vi "Launcher.vi"(8 "Error in (no error)":errorcluster) -> (0 "Error out":errorcluster)   [LabVIEW 2021]
uses:
  Controller/Controller/Controller.lvclass
  C:/Program Files/National Instruments/LabVIEW 2021/vi.lib/ActorFramework/Actor/Actor.lvclass
  <vilib>/ActorFramework/Actor/Actor.lvclass
panel:
  out "Status":string
  out "Slide":u8(slide) scale=0.0..100.0
  # "Image Harvest 1.0.0-beta"
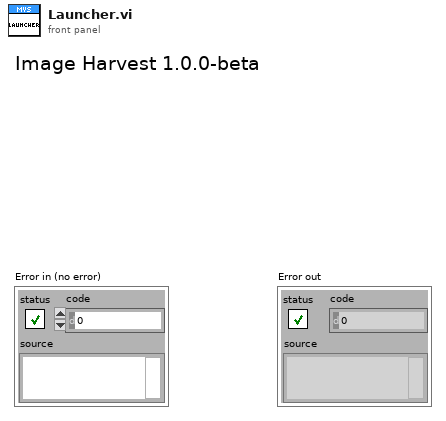
[diagram p1: front panel]
types:
  T1 = enum16{"Poll", "Initialize", "Check License", "Launch Main", "Force Stop", "Error", "Exit"}
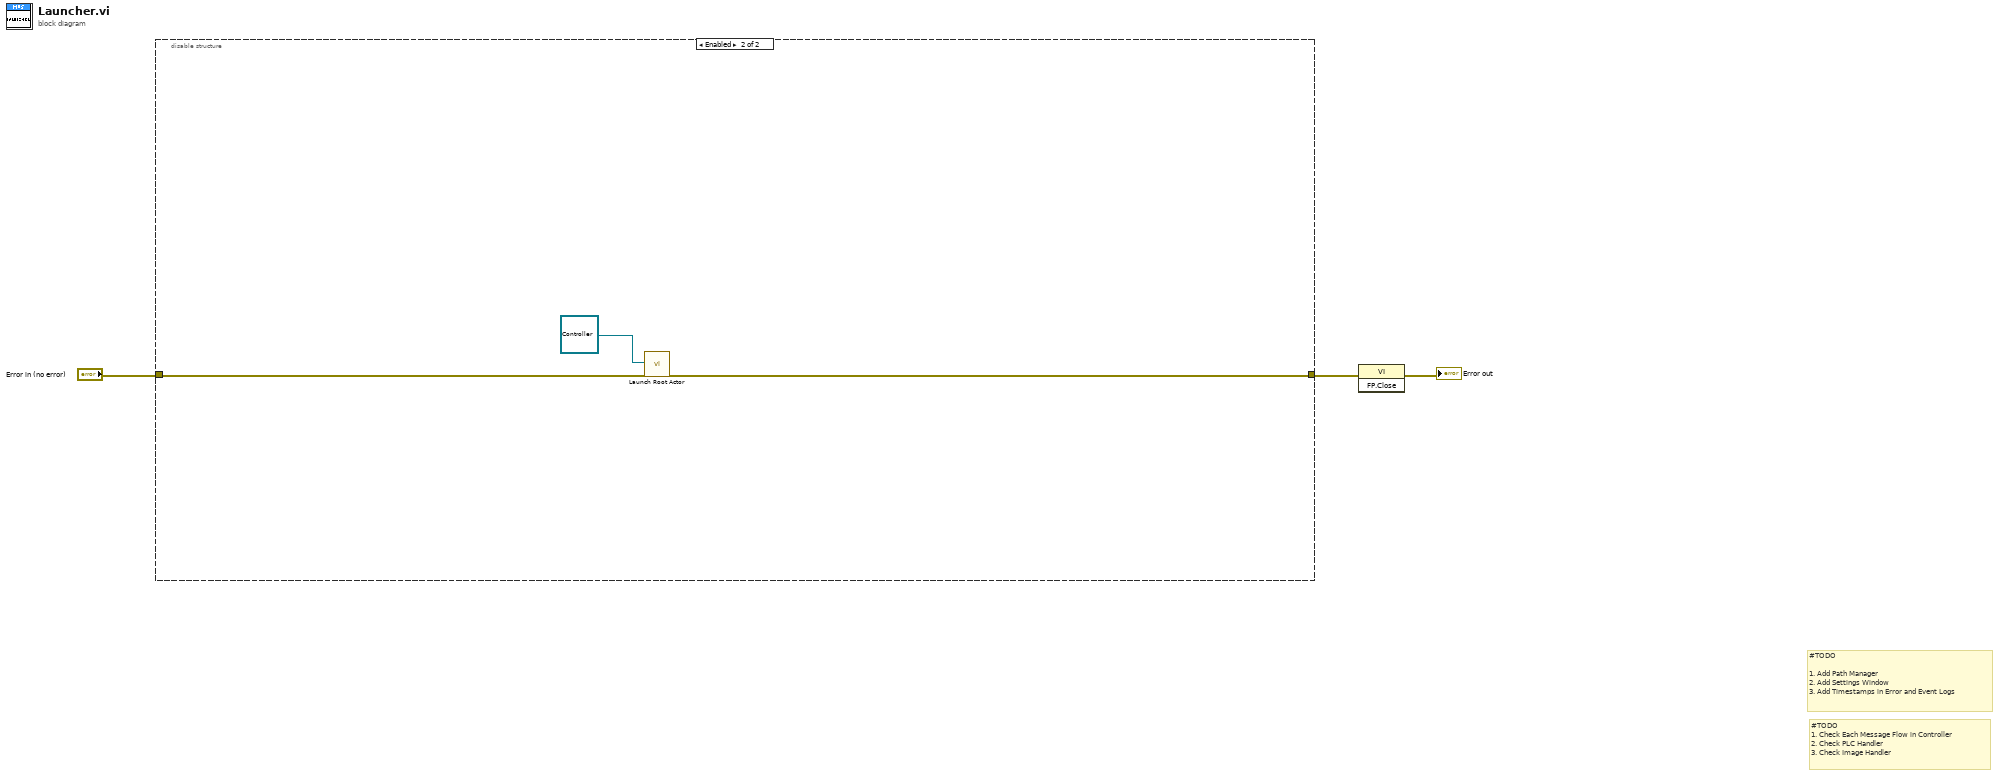
[diagram p0: block diagram]
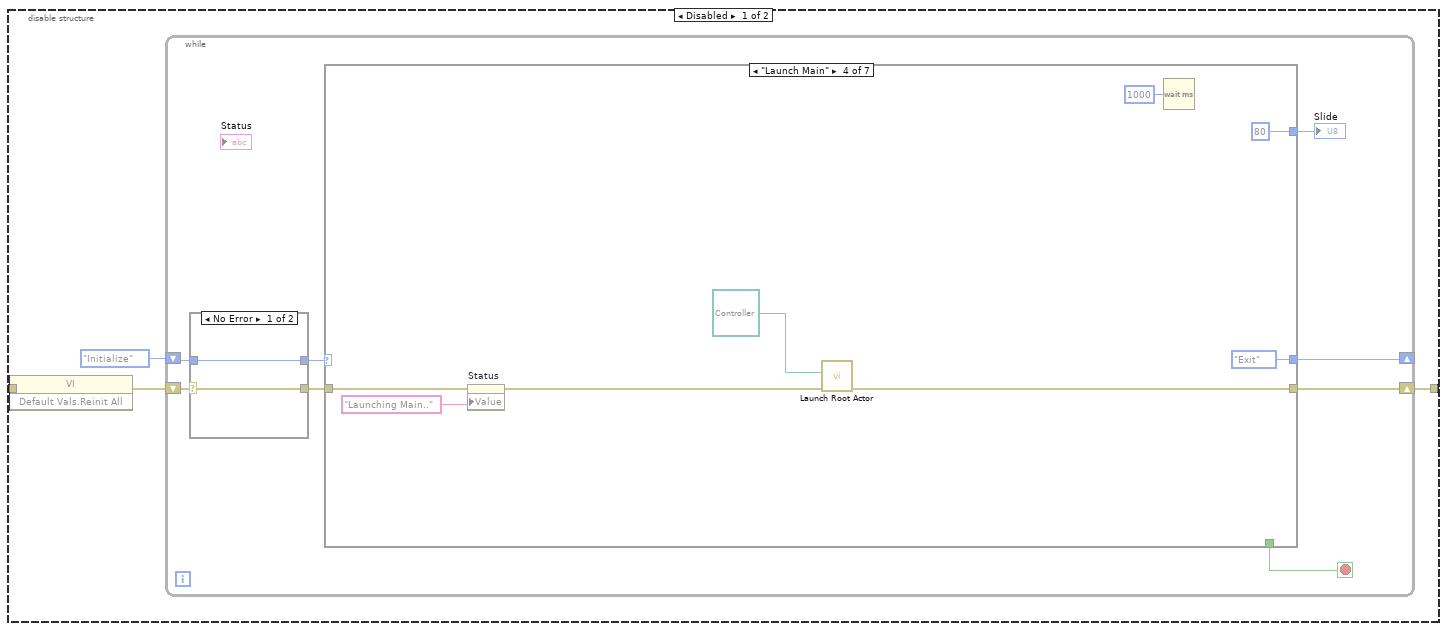
[diagram p2: hidden frame]
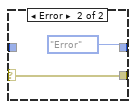
[diagram p3: hidden frame]
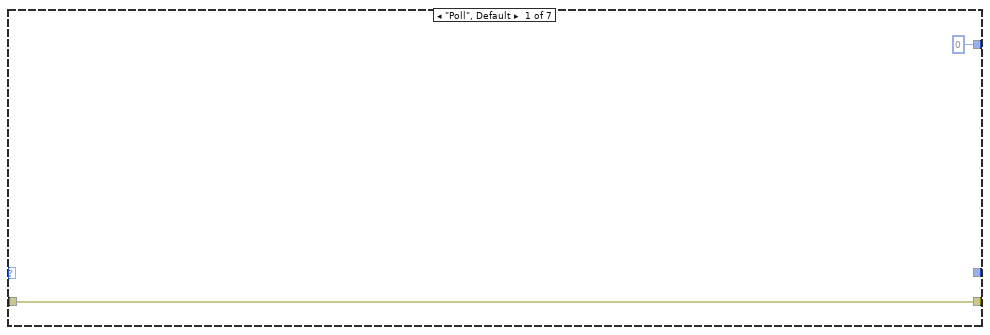
[diagram p4: hidden frame]
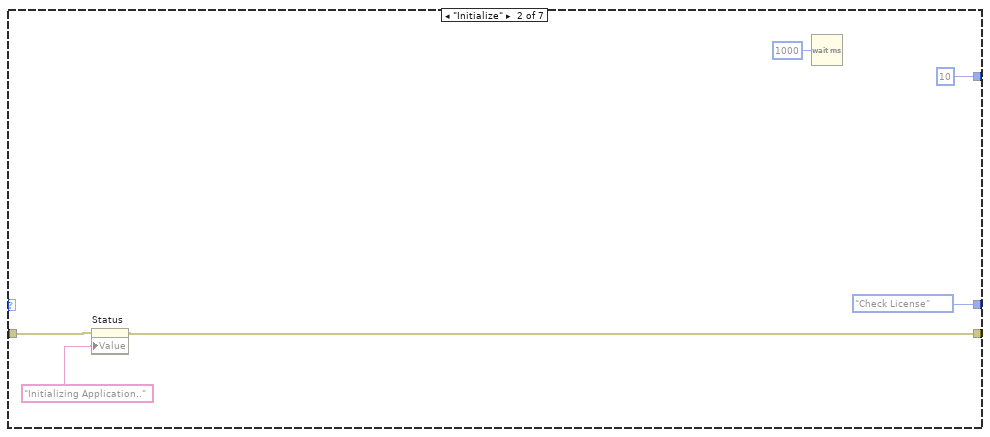
[diagram p5: hidden frame]
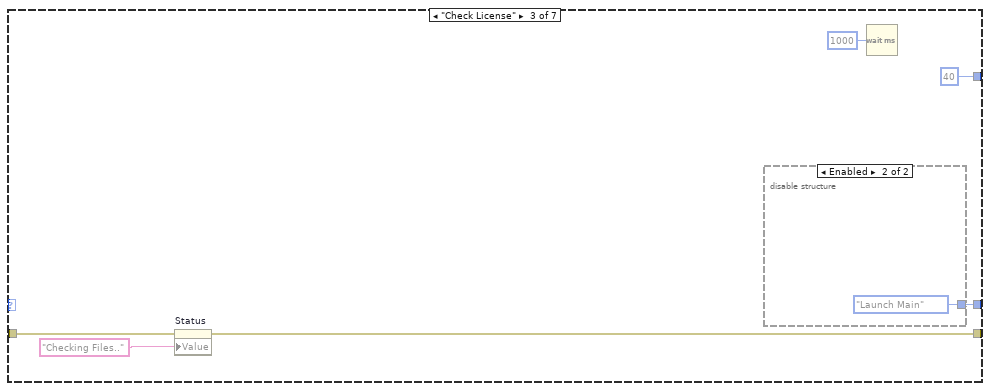
[diagram p6: hidden frame]
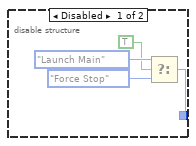
[diagram p7: hidden frame]
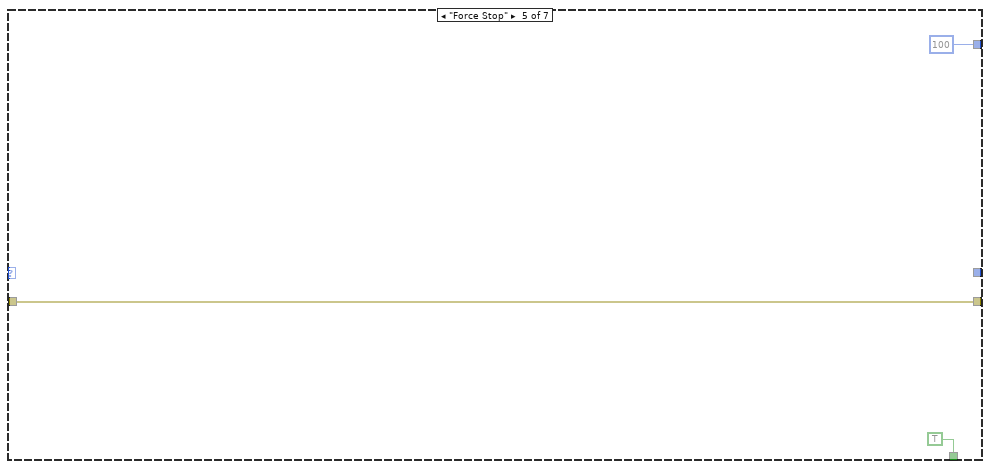
[diagram p8: hidden frame]
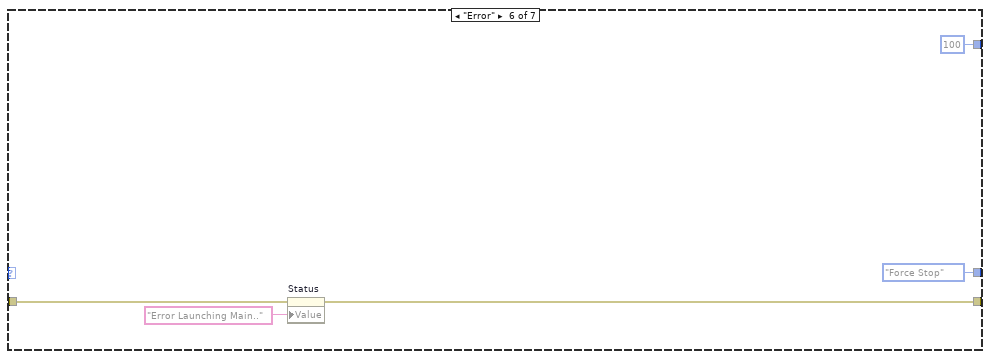
[diagram p9: hidden frame]
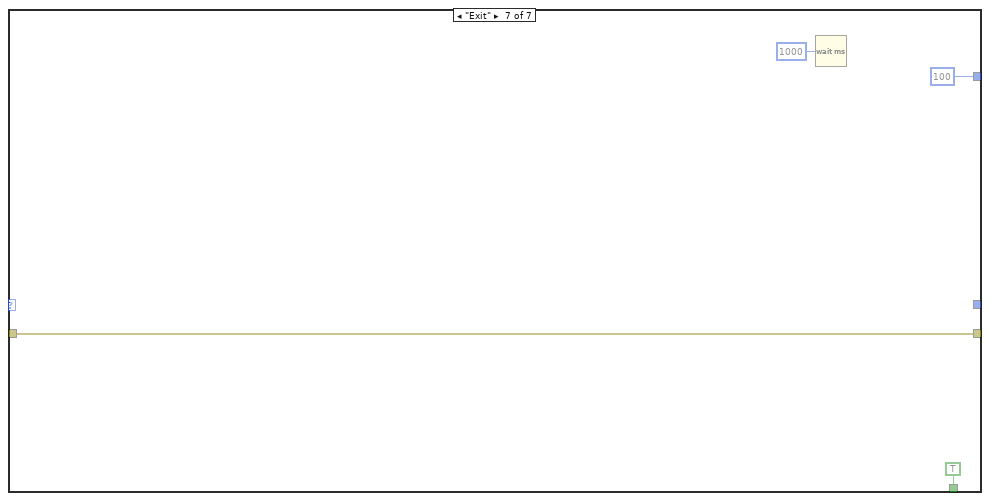
[diagram p10: hidden frame]
diagram:
  # "#TODO\n1. Check Each Message Flow in Controller\n2. Check PLC Handler\n3. Check Image Handler"
  # "#TODO\n\n1. Add Path Manager\n2. Add Settings Window\n3. Add Timestamps in Error and Event Logs"
  n1 = disable-structure shown="Enabled" {
    disable-tunnel: "Error in (no error)" -> [w6 w60]
    disable-tunnel: [w4 w59] -> w2
    frame Disabled {
      n2 = invoke class="VI" method="Default Vals.Reinit All"(error in=w6) -> (error out=w5:errorcluster)  [unwired: 2 in, 2 out]
      n3 = while {
        shift-right: [w10] -> _
        shift-left: T1."Initialize" -> [w12]
        shift-right: [w15] -> w4
        shift-left: w5 -> [w14]
        stop <- w9 stop-if-true
        n4 = case shown="No Error" w14 {
          selector: w14 -> [w17 w19]
          tunnel: [w17 w19] -> w13
          tunnel: [w16 T1."Error"] -> w11
          tunnel: w12 -> [w16 _]
          frame No Error {
          }
          frame Error {
          }
        }
        n5 = case shown="\"Launch Main\"" w11 {
          tunnel: w13 -> [w21 w24 w29 w42 w49 w52 w58]
          tunnel: [w21 w23 w28 w46 w49 w51 w58] -> w15
          tunnel: [_ T1."Check License" w33 T1."Exit" _ T1."Force Stop" _] -> w10
          tunnel: [_ _ _ _ TRUE _ TRUE] -> w9
          tunnel: [u8 0 u8 10 u8 40 u8 80 u8 100 u8 100 u8 100] -> w8
          frame "Poll", Default {
          }
          frame "Initialize" {
            n6 = property on="Status" class="Str"(error in=w24, "Value"="Initializing Application.." ("Caption.Text")) -> (error out=w23:errorcluster)  [unwired: 1 in, 1 out]
            n7 = Wait (ms)(milliseconds to wait=u32 1000) -> ()  [unwired: 1 out]
          }
          frame "Check License" {
            n8 = property on="Status" class="Str"(error in=w29, "Value"="Checking Files.." ("Caption.Text")) -> (error out=w28:errorcluster)  [unwired: 1 in, 1 out]
            n9 = disable-structure shown="Enabled" {
              disable-tunnel: [w37 T1."Launch Main"] -> w33
              frame Disabled {
                n10 = Select(t=T1."Launch Main", s=TRUE, f=T1."Force Stop") -> (s? t:f=w37:T1)
              }
              frame Enabled {
              }
            }
            n11 = Wait (ms)(milliseconds to wait=u32 1000) -> ()  [unwired: 1 out]
          }
          frame "Launch Main" {
            n12 = property on="Status" class="Str"(error in=w42, "Value"="Launching Main.." ("Caption.Text")) -> (error out=w41:errorcluster)  [unwired: 1 in, 1 out]
            n13 = call <vilib>:"Launch Root Actor.vi"("error in (no error)"=w41, "Actor"=refnum<class "Controller.lvclass"> refnum ("Controller.lvlib:Controller.lvclass")) -> ("error out"=w46:errorcluster)  [unwired: 8 in, 1 out]
            n14 = Wait (ms)(milliseconds to wait=u32 1000) -> ()  [unwired: 1 out]
          }
          frame "Force Stop" {
          }
          frame "Error" {
            n15 = property on="Status" class="Str"(error in=w52, "Value"="Error Launching Main.." ("Caption.Text")) -> (error out=w51:errorcluster)  [unwired: 1 in, 1 out]
          }
          frame "Exit" {
            n16 = Wait (ms)(milliseconds to wait=u32 1000) -> ()  [unwired: 1 out]
          }
        }
        "Slide" <- w8
      }
    }
    frame Enabled {
      n17 = call <vilib>:"Launch Root Actor.vi"("error in (no error)"=w60, "Actor"=refnum<class "Controller.lvclass"> refnum ("Controller.lvlib:Controller.lvclass")) -> ("error out"=w59:errorcluster)  [unwired: 8 in, 1 out]
    }
  }
  n18 = invoke class="VI" method="FP.Close"(error in=w2) -> (error out=→"Error out":errorcluster)  [unwired: 2 in, 2 out]
